vi "getChipSize.vi"(6 "Delay between send and receive [ms]":i32=100, 8 "error in (no error)":errorcluster, 11 "CCD in":refnum<class "CCD.lvclass">) -> (0 "error out":errorcluster, 1 "chip size, y":i32, 2 "chip size, x":i32, 3 "CCD out":refnum<class "CCD.lvclass">)   [LabVIEW 2023, in "CCD.lvclass"]
doc: "Returns the chip sensor’s pixel width and height size.\n\nReturn Results:\n\nresults description\nx Integer. Chip sensor's x size in pixels (width)\ny Integer. Chip sensor's y size in pixels (height)"
uses:
  CCD.lvclass
  CCD.lvclass/CCD.ctl
  acd18d44-655d-42a0-b073-c3a6adbe6448.vi
  Chipsize.ctl
  91ff1499-e288-40ed-a9bd-2102f7a68490.vi
  GenericDevice/GenericDevice.lvclass
panel:
  # "Connector Pane"
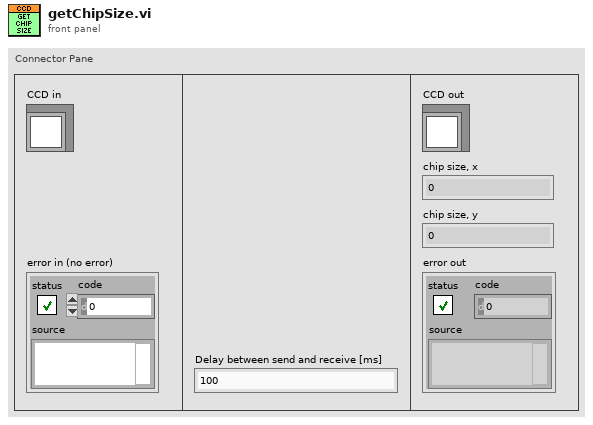
[diagram p1: front panel]
types:
  T1 = typedef "CCD.lvclass/Chipsize.ctl" = cluster{"x":i32, "y":i32}
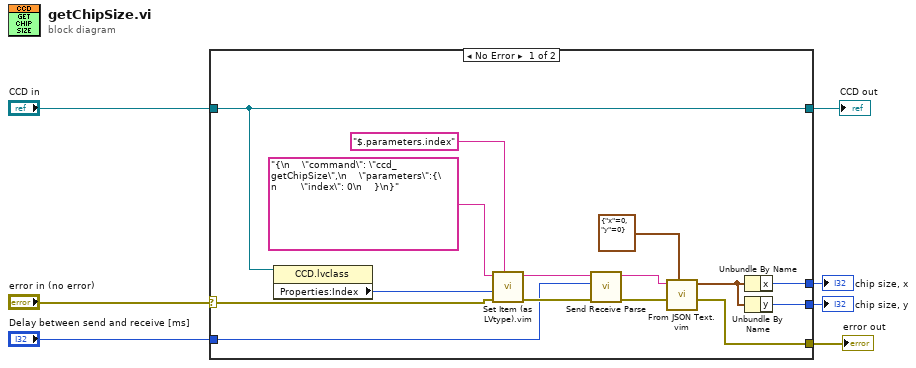
[diagram p0: block diagram]
diagram:
  n1 = case shown="No Error" "error in (no error)" {
    selector: "error in (no error)" -> [w18 w24]
    tunnel: [w17 w24] -> w6
    tunnel: [w20 w23] -> w4
    tunnel: "CCD in" -> [w20 w23]
    tunnel: [w11 _] -> w3
    tunnel: [w10 _] -> w2
    tunnel: "Delay between send and receive [ms]" -> [w9 _]
    frame No Error {
      n2 = property class="CCD.lvclass"(reference=w20) -> ("Properties:Index"=w19:i32)  [unwired: 1 in, 2 out]
      n3 = call "Set Item (as LVtype).vim"("$Path or Item Name"="$.parameters.index", "error in (no error)"=w18, "Anything"=w19, "JSON"="{\n    \"command\": \"ccd_getChipSize\",\n    \"parameters\":{\n        \"index\": 0\n    }\n}") -> ("error out"=w14:errorcluster, "<JSON>"=w8:string)  [unwired: 4 in, 1 out]
      n4 = call "Send Receive Parse.vi"("error in"=w14, "Delay between send and receive [ms]"=w9, "<JSON>"=w8) -> ("error out"=w13:errorcluster, "results-JSON string"=w15:string)  [unwired: 6 in, 1 out]
      n5 = call "From JSON Text.vim"("Data Type and Default Value"=T1 {"x"=0, "y"=0} ("Chipsize"), "error in (no error)"=w13, "JSON"=w15) -> ("error out"=w17:errorcluster, "Data out"=w12:T1)  [unwired: 7 in]
      n6 = Unbundle By Name(w12) -> ("x"=w11:i32)
      n7 = Unbundle By Name(w12) -> ("y"=w10:i32)
    }
    frame Error {
    }
  }
  "error out" <- w6
  "CCD out" <- w4
  "chip size, x" <- w3
  "chip size, y" <- w2
